vi "CurveTrace_Single.vi"(0 "Test Params Cluster":T1={"Test Freq. (Hz)"=100.0, "Output Signal Amplitude\nVolts Pk"=5.0, "Sampling Time (s)"=0.01, "Sampling Rate (Hz)"=250000.0, "Output Channel"="PXI1Slot2/ao0", "Current Channel"="PXI1Slot2/ai1", "Voltage Channel"="PXI1Slot2/ai2", "Trigger Channel"="/PXI1Slot2/ao/StartTrigger", "Number of runs"=5, "BaseGateBias Channel"="PXI1Slot2/ao1"}) -> ()   [LabVIEW 2022 SP3]
uses:
  <vilib>/Analysis/1siggen.llb/Ramp Pattern by Samples.vi
  <vilib>/Analysis/NI_AALBase.lvlib
panel:
  in  "start":dbl=2.5 format="%0.2f"
  in  "end":dbl=4.0 format="%0.2f"
  in  "samples":i32=50
  in  "offset":dbl format="%#_13g"
  out "XY Graph":cluster{"Y":dbl[], "Y":dbl[]}[](graph)
  in  "Tab Control":enum32{"Inputs", "Outputs", "Additional Plots"}(tab)
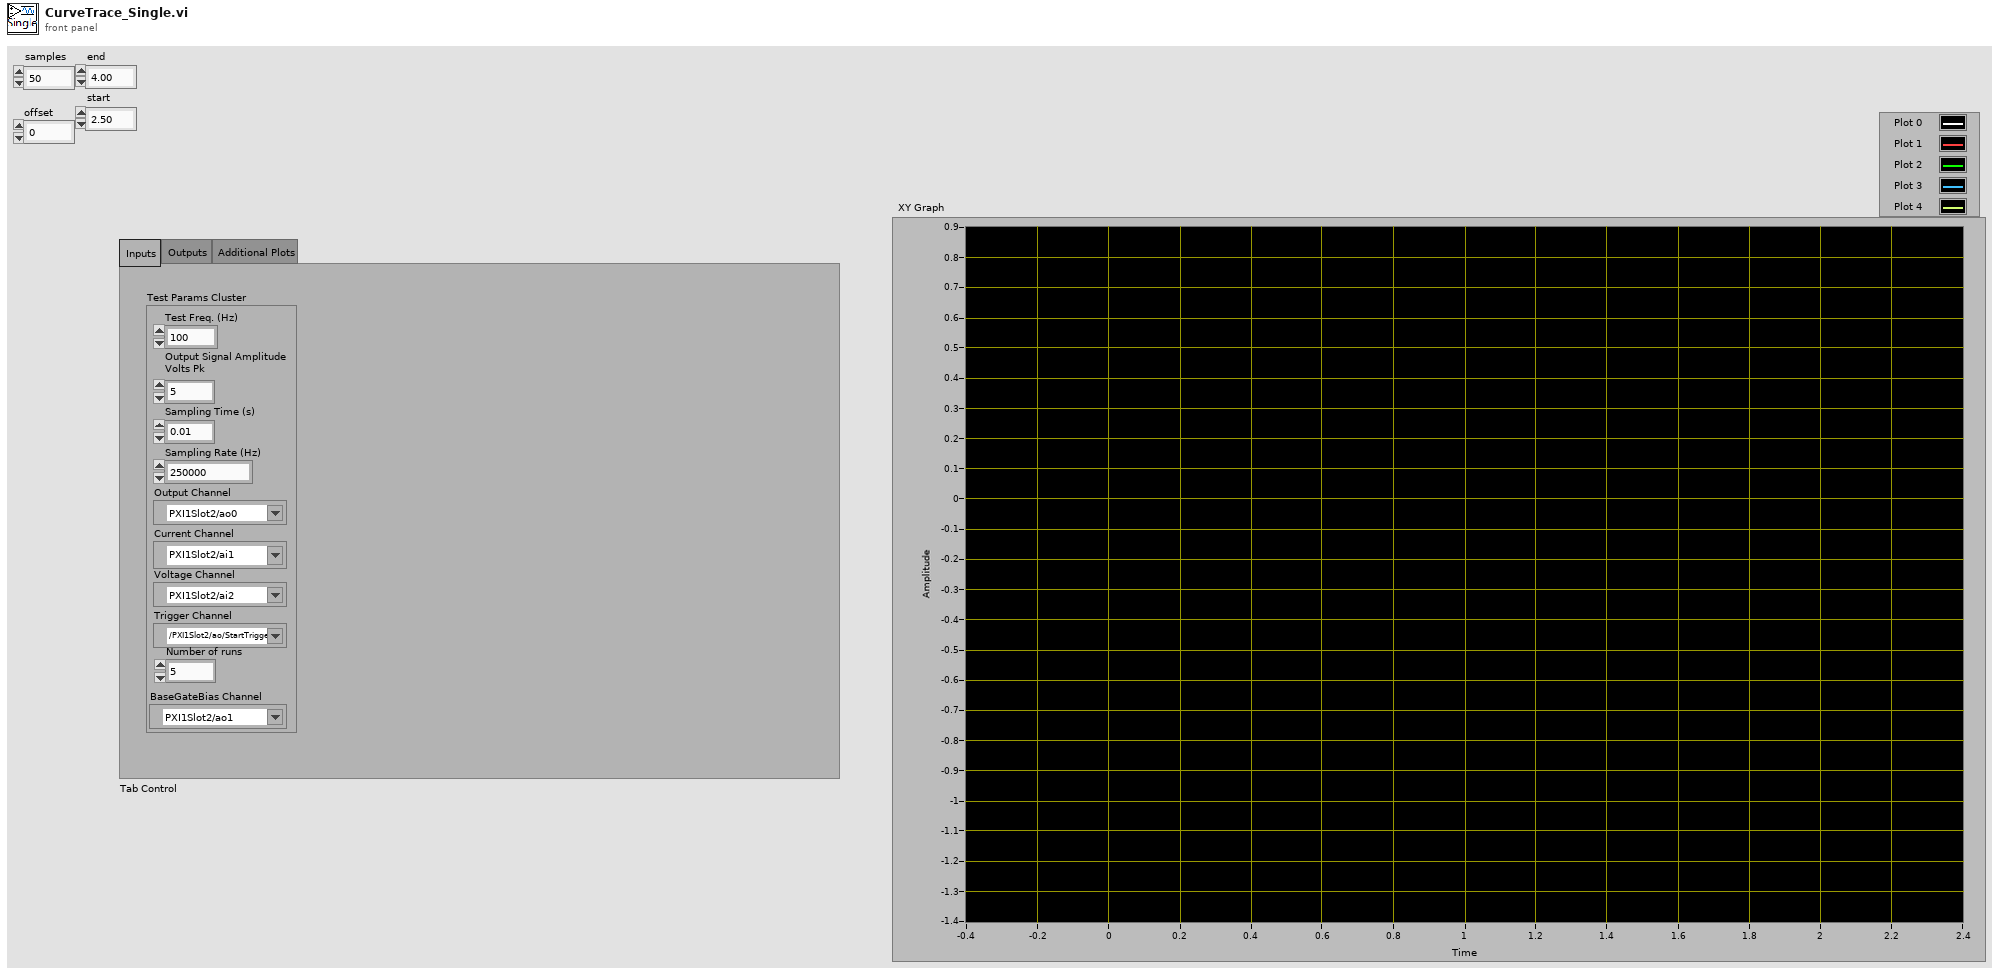
[diagram p1: front panel]
types:
  T1 = cluster{"Test Freq. (Hz)":dbl, "Output Signal Amplitude\nVolts Pk":dbl, "Sampling Time (s)":dbl, "Sampling Rate (Hz)":dbl, "Output Channel":tag, "Current Channel":tag, "Voltage Channel":tag, "Trigger Channel":tag, "Number of runs":i32, "BaseGateBias Channel":tag}
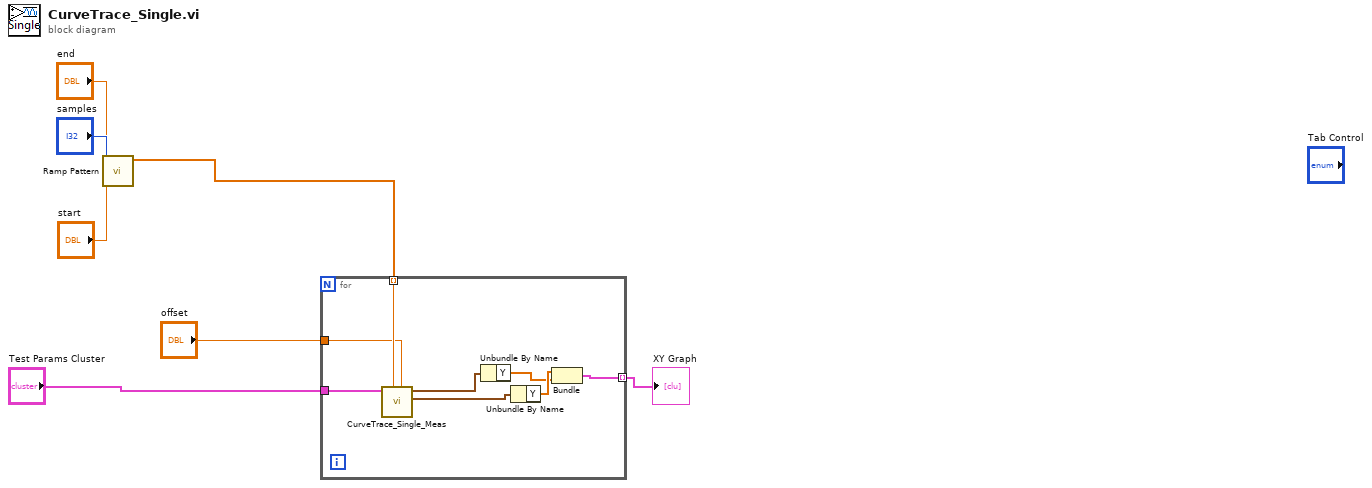
[diagram p0: block diagram]
diagram:
  n1 = call-poly <vilib>:"Ramp Pattern.vi"("start"="start", "end"="end", "samples"="samples") -> ("Ramp Pattern"=w4:dbl[])  [unwired: 7 in, 1 out]
  n2 = for {
    tunnel: "Test Params Cluster" -> [w15]
    tunnel: w4 -> [w10] mode=indexing
    tunnel: [w9] -> w6 mode=indexing
    tunnel: "offset" -> [w8]
    n3 = call "CurveTrace_Single_Meas.vi"("offset"=w8, "Base Gate Bias Value"=w10, "Test Params Cluster"=w15) -> ("Time domain Current"=w13:waveform(dbl), "Time domain Voltage"=w14:waveform(dbl))  [unwired: 5 in, 2 out]
    n4 = Unbundle By Name(w14) -> ("Y"=w11:dbl[])
    n5 = Unbundle By Name(w13) -> ("Y"=w12:dbl[])
    n6 = Bundle("Y"=w12, "Y"=w11) -> (w9:cluster{"Y":dbl[], "Y":dbl[]})  [unwired: 1 in]
  }
  "XY Graph" <- w6
